vi "DrivePath.vi"(2 "Parameter String":string, 3 "Reinit":bool) -> (0 "Path Follower Error":errorcluster, 1 "Increment":bool)   [LabVIEW 2019]
doc: "A pure-pursuit path-following algorithm configured for a swerve drive. Feed-forward and feed-back controllers are combined to produce unitless drive commands. This VI is designed to integrated with the FRC 4265 Autonomous Path Planner. The Search Window can be specified in seconds - longer search windows are more robust to recovering from large deviations from the path but may cause the robot to \"jump\" ahead when following tight loops or turns. The Look-Ahead Time specifies the furthest ahead the pursuit point can be.\n\nParameters:\n1. acceptable distance error --> (in) [0,614.25]\n2. acceptable angle error --> (deg) [0,180]\n3. path follow timeout --> (ms) [0,15000] set to -1 for no timeout\n3. name of the autonomous path\n4. specifiy whether or not the robot can add a suffix to the selected path name {normal,robot_suffix}"
uses:
  sensors.vi
  dscommands.vi
  autoninfo.vi
  SafeParser_Float.vi
  SafeParser_Integer.vi
  5c80b45a-8b82-4ca3-a7a6-7ac929992d21.vi
  SafeParser_String.vi
panel:
  out "PID Strafe":T1(graph)
  in  "PID Tuning Strafe":T2={"Kp"=0.02, "Ki"=0.0, "Kd"=0.0, "N-Diff"=10, "N-Int"=10, "Int Error Window"=5.0, "Max Ouput"=1.0, "Min Output"=-1.0} {"Int Error Window" min=0.0; "N-Int" min=2; "N-Diff" min=2; "Kd" min=0.0; "Ki" min=0.0; "Kp" min=0.0}
  out "PID Heading":T1(graph)
  in  "PID Tuning Heading":T2={"Kp"=0.006, "Ki"=0.0, "Kd"=0.0, "N-Diff"=10, "N-Int"=10, "Int Error Window"=30.0, "Max Ouput"=1.0, "Min Output"=-1.0} {"Int Error Window" min=0.0; "N-Int" min=2; "N-Diff" min=2; "Kd" min=0.0; "Ki" min=0.0; "Kp" min=0.0}
  out "Path and Robot Pose":cluster{dbl[], dbl[]}[](graph)
  in  "Plot":bool
  in  "Max Look-Ahead Time (s)":dbl=0.5
  in  "Search Window (s)":dbl=2.0
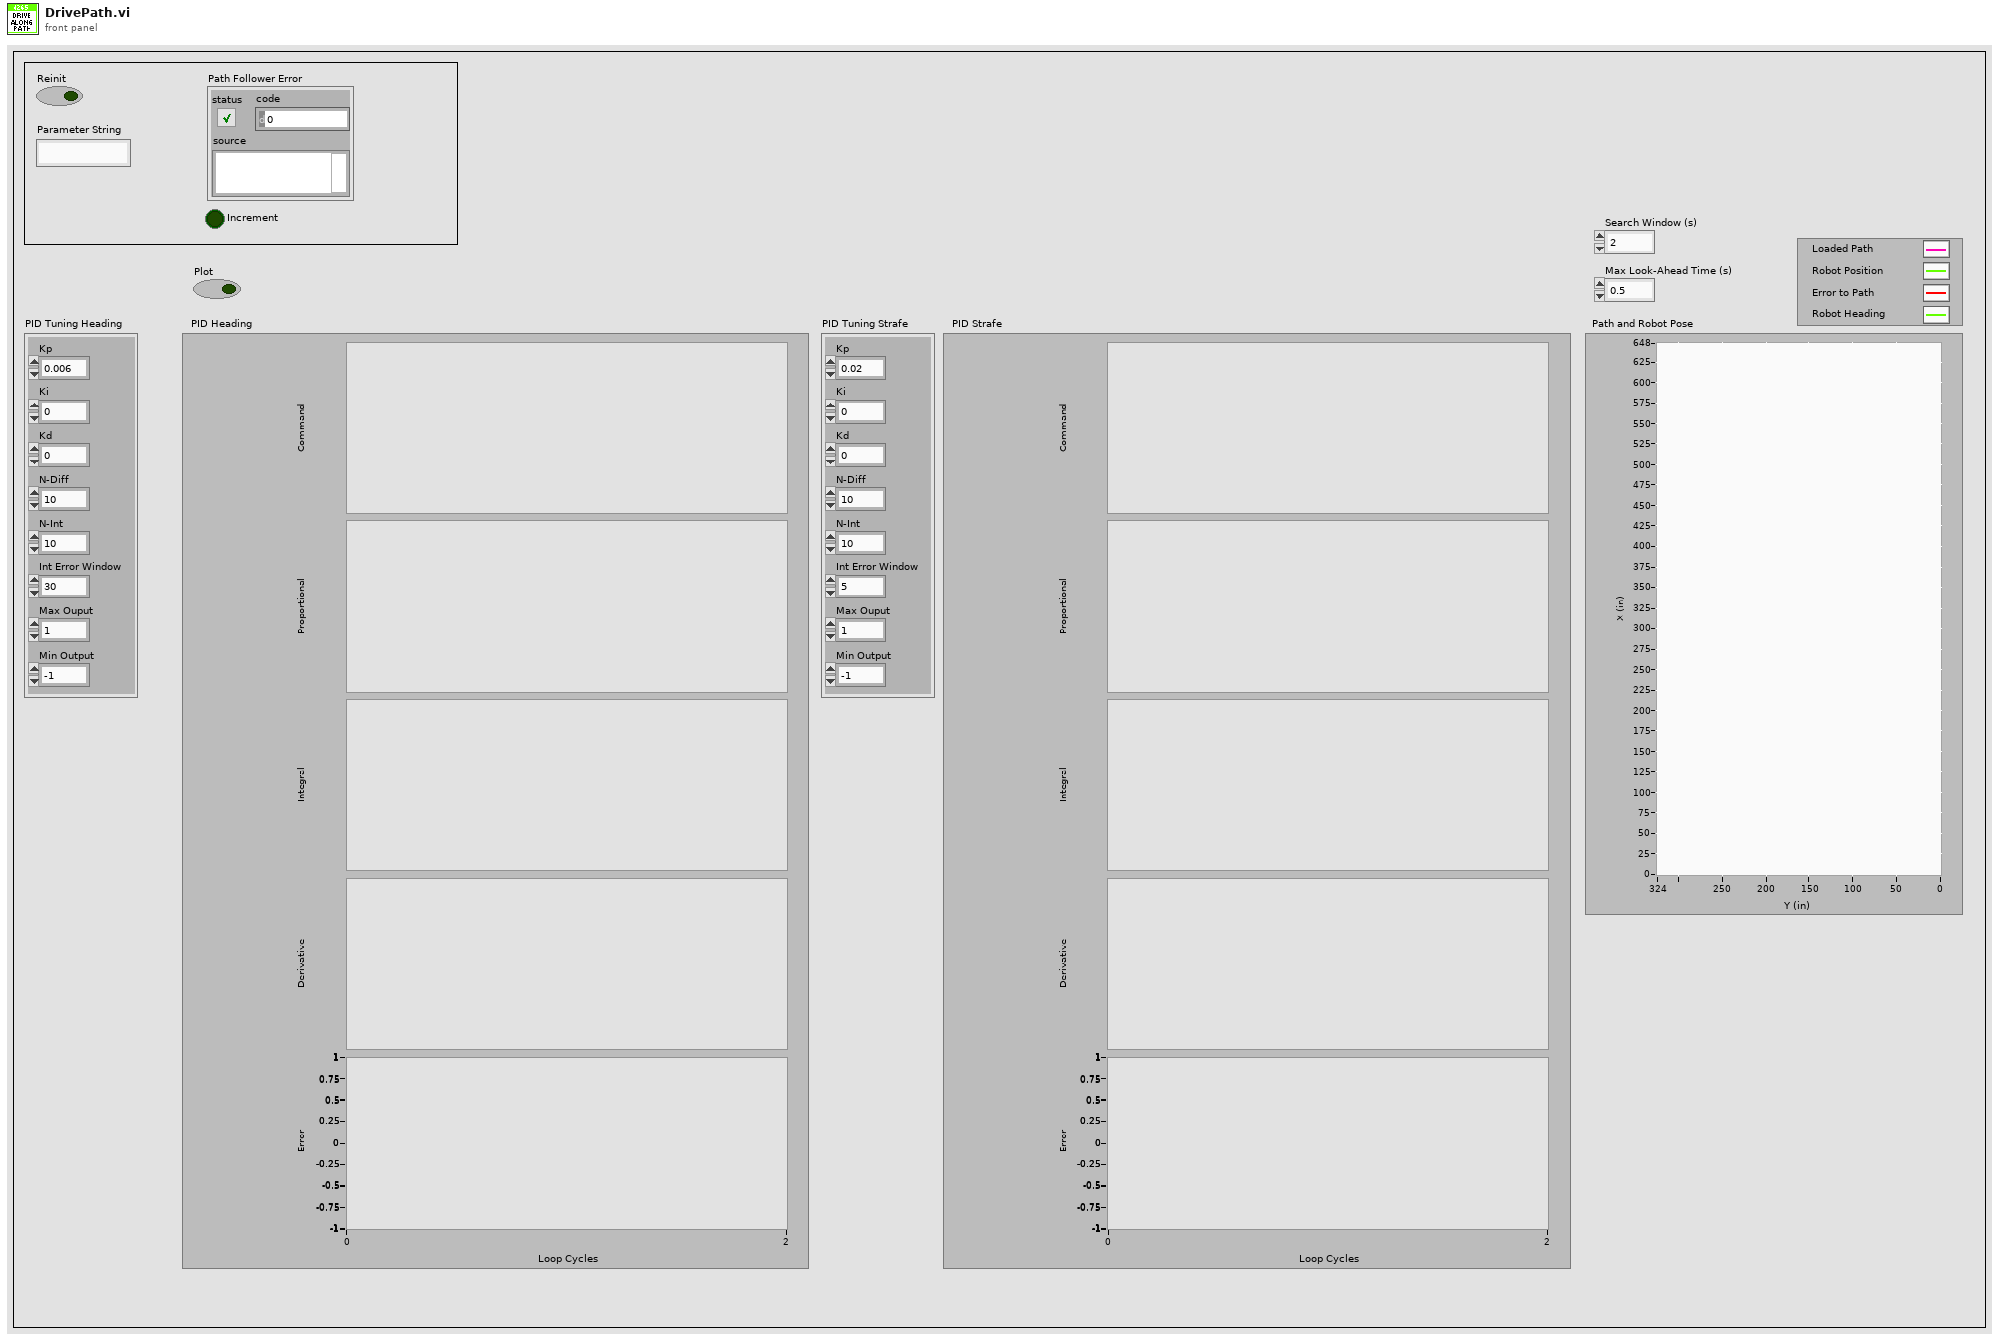
[diagram p1: front panel]
types:
  T1 = cluster{"Command":dbl, "Proportional":dbl, "Integral":dbl, "Derivative":dbl, "Goal":dbl}
  T2 = cluster{"Kp":dbl, "Ki":dbl, "Kd":dbl, "N-Diff":i32, "N-Int":i32, "Int Error Window":dbl, "Max Ouput":dbl, "Min Output":dbl}
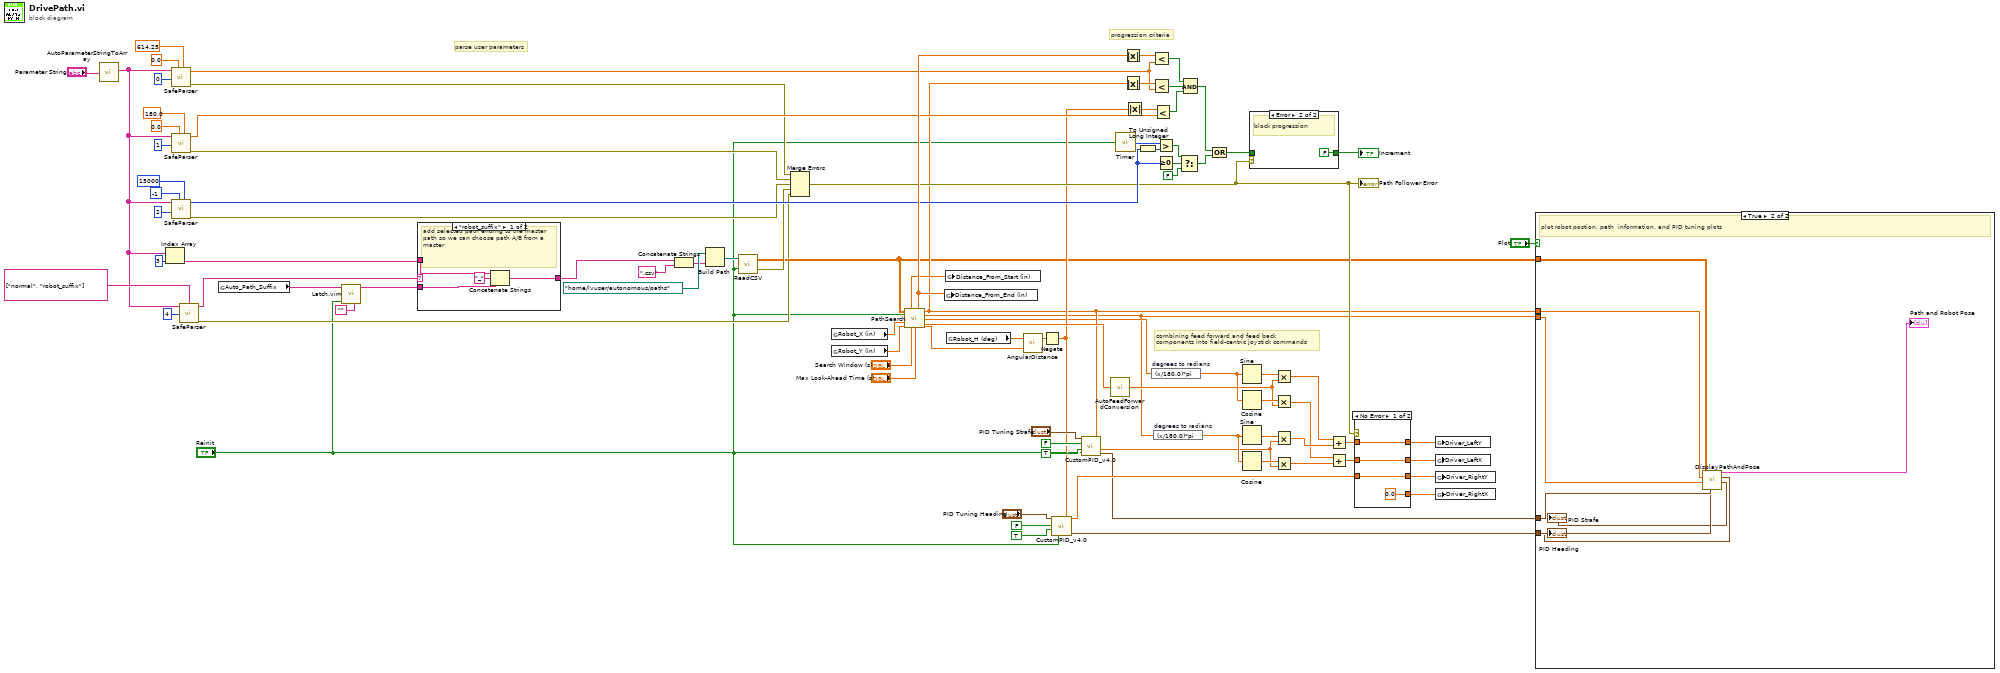
[diagram p0: block diagram]
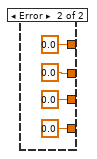
[diagram p5: hidden frame]
diagram:
  # "parse user parameters"
  # "progression criteria"
  # "combining feed forward and feed back\ncomponents into field-centric joystick commands"
  n1 = call "AutoParameterStringToArray.vi"("Parameter String"="Parameter String") -> ("Parsed Parameters"=w19:string[])
  n2 = Index Array(array=w19, index=3) -> (element=w22:string)
  n3 = call-poly "SafeParser.vi"("Maximum"=614.25, "Minimum"=0.0, "Array Index"=0 ("Parameter Index"), "String Array"=w19) -> ("Error Out"=w52:errorcluster, "Typecast  Value"=w60:dbl)  [unwired: 6 in]
  n4 = call-poly "SafeParser.vi"("Maximum"=180.0, "Minimum"=0.0, "Array Index"=1 ("Parameter Index"), "String Array"=w19) -> ("Error Out"=w53:errorcluster, "Typecast  Value"=w57:dbl)  [unwired: 6 in]
  n5 = call-poly "SafeParser.vi"("Maximum"=15000, "Minimum"=-1, "Array Index"=2 ("Parameter Index"), "String Array"=w19) -> ("Error Out"=w54:errorcluster, "Typecast  Value"=w65:i32)  [unwired: 6 in]
  n6 = call-poly "SafeParser.vi"("Allowed Values"=string[] ["normal", "robot_suffix"], "Array Index"=4, "String Array"=w19) -> ("Error Out"=w18:errorcluster, "Typecast Value"=w20:string)  [unwired: 7 in]
  n7 = global read "autoninfo.vi" "Auto_Path_Suffix"() -> (w4:string)
  n8 = call "Latch.vim"("Default Value"="", "Latch Signal"="Reinit", "Latch Value"=w4) -> ("Latched"=w1:string)  [unwired: 8 in]
  n9 = case shown="\"robot_suffix\"" w20 {
    tunnel: w22 -> [w96 w97]
    tunnel: [w95 w97] -> w21
    tunnel: w1 -> [w94 _]
    frame "robot_suffix" {
      # "add selected path ending to the master \npath so we can choose path A/B from a master"
      n10 = Concatenate Strings(w96, "_" ("string"), w94) -> (w95:string)
    }
    frame "normal", Default {
    }
  }
  n11 = Concatenate Strings(w21, ".csv" ("string")) -> (w85:string)
  n12 = Build Path(base path=path "/home/lvuser/autonomous/paths" ("path"), name or relative path=w85) -> (appended path=w91:path)
  n13 = call "ReadCSV.vi"("Reinit"="Reinit", "File Path (.csv)"=w91) -> ("File Open Eror"=w55:errorcluster, "Data (index by row)"=w27:dbl[][])
  n14 = Merge Errors(w52, w53, w54, w55, w18) -> (w56:errorcluster)
  "Path Follower Error" <- w56
  n15 = global read "sensors.vi" "Robot_X (in)"() -> (w90:dbl)
  n16 = global read "sensors.vi" "Robot_Y (in)"() -> (w89:dbl)
  n17 = call "PathSearch.vi"("Path"=w27, "Reint"="Reinit", "Robot X (in)"=w90, "Robot Y (in)"=w89, "Search Window (s)"="Search Window (s)", "Look-Ahead Time (s)"="Max Look-Ahead Time (s)") -> ("Distance from Start (in)"=w78:dbl, "Distance from End (in)"=w79:dbl, "Feed Back Distance Error (in)"=w33:dbl, "Feed Back Pointing Angle (deg)"=w12:dbl, "Feed Forward Pointing Angle (deg)"=w17:dbl, "Feed Forward Velocity (in/s)"=w80:dbl, "Robot Heading Goal (deg)"=w68:dbl)  [unwired: 3 in]
  n18 = global write "autoninfo.vi" "Distance_From_End (in)"(w79) -> ()
  n19 = global write "autoninfo.vi" "Distance_From_Start (in)"(w78) -> ()
  n20 = global read "sensors.vi" "Robot_H (deg)"() -> (w40:dbl)
  n21 = call "AngularDistance.vi"("Goal Angle (deg) [0,360]"=w68, "Current Angle (deg) [-Inf,+Inf]"=w40) -> ("Signed Angular Distance (deg) [-180,+180]"=w38:dbl)  [unwired: 1 out]
  n22 = Negate(x=w38) -> (-x=w37:dbl)
  n23 = call "CustomPID_v4.0.vi"("PID Tuning Parameters"="PID Tuning Heading", "Custom Error Calculation"=w37, "Reset on Goal Change ?"=FALSE, "Use Custom Error Calculation ?"=TRUE, "Reinit"="Reinit") -> ("Command"=w48:dbl, "Controller Summary"=w36:T1)  [unwired: 7 in, 2 out]
  n24 = call "CustomPID_v4.0.vi"("PID Tuning Parameters"="PID Tuning Strafe", "Custom Error Calculation"=w33, "Reset on Goal Change ?"=FALSE, "Use Custom Error Calculation ?"=TRUE, "Reinit"="Reinit") -> ("Command"=w11:dbl, "Controller Summary"=w43:T1)  [unwired: 7 in, 2 out]
  n25 = call "AutoFeedForwardConversion.vi"("Target Velocity (in/s)"=w80) -> ("Equivalent Joystick Command (ul)"=w16:dbl)
  n26 = call "Timer.vi"("Reset Timer"="Reinit") -> ("Time (ms)"=w69:u32)
  n27 = Absolute Value(x=w79) -> (abs(x)=w70:dbl)
  n28 = Absolute Value(x=w33) -> (abs(x)=w71:dbl)
  n29 = Absolute Value(x=w37) -> (abs(x)=w77:dbl)
  n30 = To Unsigned Long Integer(number=w65) -> (unsigned 32bit integer=w75:u32)
  n31 = expression code="(x/180.0)*pi" "degrees to radians"(w17) -> (w83:dbl)
  n32 = Less?(x=w70, y=w60) -> (x < y?=w30:bool)
  n33 = Less?(x=w71, y=w60) -> (x < y?=w31:bool)
  n34 = Less?(x=w77, y=w57) -> (x < y?=w32:bool)
  n35 = expression code="(x/180.0)*pi" "degrees to radians"(w12) -> (w15:dbl)
  n36 = Greater?(x=w69, y=w75) -> (0:w73:bool)
  n37 = Greater Or Equal To 0?(x=w65) -> (x >= 0?=w74:bool)
  n38 = Select(t=w73, s=w74, f=FALSE) -> (s? t:f=w28:bool)
  n39 = Compound Arithmetic op=AND(w30, w31, w32) -> (w29:bool)
  n40 = Compound Arithmetic op=OR(w29, w28) -> (w76:bool)
  n41 = Sine(x=w83) -> (sin(x)=w82:dbl)
  n42 = Cosine(x=w83) -> (cos(x)=w81:dbl)
  n43 = Sine(x=w15) -> (sin(x)=w14:dbl)
  n44 = Cosine(x=w15) -> (cos(x)=w13:dbl)
  n45 = case shown="Error" w56 {
    tunnel: [w98 FALSE] -> w86
    tunnel: w76 -> [w98 _]
    frame No Error {
      # "allow progression"
    }
    frame Error {
      # "block progression"
    }
  }
  "Increment" <- w86
  n46 = Multiply(x=w82, y=w16) -> (x*y=w10:dbl)
  n47 = Multiply(x=w81, y=w16) -> (x*y=w8:dbl)
  n48 = Multiply(x=w14, y=w11) -> (x*y=w9:dbl)
  n49 = Multiply(x=w13, y=w11) -> (x*y=w7:dbl)
  n50 = Add(x=w10, y=w9) -> (x+y=w6:dbl)
  n51 = Add(x=w8, y=w7) -> (x+y=w5:dbl)
  n52 = case shown="No Error" w56 {
    tunnel: [w100 0.0] -> w35
    tunnel: [w103 0.0 ("upper limit")] -> w84
    tunnel: [w101 0.0] -> w34
    tunnel: w48 -> [w103 _]
    tunnel: [0.0 0.0] -> w39
    tunnel: w6 -> [w101 _]
    tunnel: w5 -> [w100 _]
    frame No Error {
    }
    frame Error {
    }
  }
  n53 = global write "dscommands.vi" "Driver_LeftY"(w34) -> ()
  n54 = global write "dscommands.vi" "Driver_LeftX"(w35) -> ()
  n55 = global write "dscommands.vi" "Driver_RightY"(w84) -> ()
  n56 = global write "dscommands.vi" "Driver_RightX"(w39) -> ()
  n57 = case shown="True" "Plot" {
    tunnel: w12 -> [_ w115]
    tunnel: w43 -> [_ w114]
    tunnel: w36 -> [_ w113]
    tunnel: w33 -> [_ w112]
    tunnel: w27 -> [_ w111]
    frame False {
    }
    frame True {
      # "plot robot postion, path  information, and PID tuning plots"
      n58 = call "DisplayPathAndPose.vi"("Controller Summary 2"=w114, "Controller Summary"=w113, "Feed Back Pointing Angle (deg)"=w115, "Feed Back Distance Error (in)"=w112, "Data (index by row)"=w111) -> ("PID Strafe"=→"PID Strafe":T1, "PID Heading"=→"PID Heading":T1, "Path and Robot Pose"=→"Path and Robot Pose":cluster{dbl[], dbl[]}[])  [unwired: 4 in]
    }
  }
